vi "Ravel Index.vi"(1 "Coerce (T)":bool=TRUE, 2 "ND Index":i32[](array[numeric]), 3 "Array Shape":i32[](array[numeric])) -> (0 "Flat Index":i32)   [LabVIEW 2020, in "VIM Tools.lvlib"]
uses:
  VIM Tools.lvlib
  6fbc3370-4fe2-4f23-9844-c55be6350a4c.vi
  5715f375-2f19-42b1-8971-07d7b1a35376.vi
  f35ef6e7-f3ea-4c67-be1f-69a31266ebf5.vi
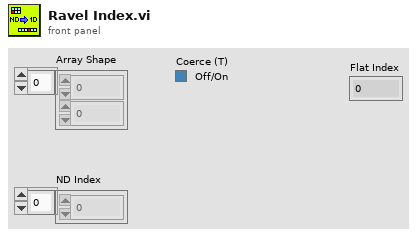
[diagram p1: front panel]
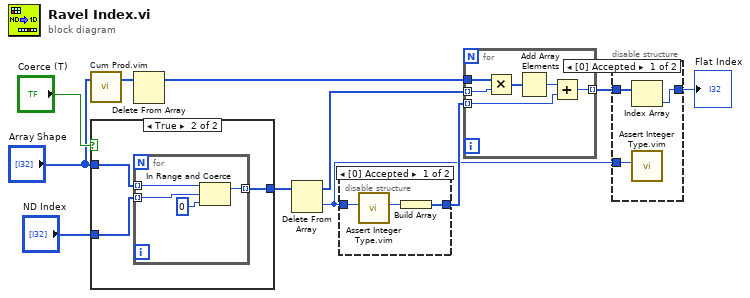
[diagram p0: block diagram]
diagram:
  n1 = call "Cum Prod.vim"("Array In"="Array Shape") -> ("Cumulated Products Out"=w10:i32[])  [unwired: 1 in, 1 out]
  n2 = case shown="True" "Coerce (T)" {
    tunnel: "ND Index" -> [w12 w15]
    tunnel: "Array Shape" -> [_ w14]
    tunnel: [w12 w13] -> w9
    frame False {
    }
    frame True {
      n3 = for {
        tunnel: w14 -> [w18] mode=indexing
        tunnel: w15 -> [w19] mode=indexing
        tunnel: [w16] -> w13 mode=indexing
        n4 = In Range and Coerce(upper limit=w18, x=w19, lower limit=0) -> (coerced(x)=w16:i32)  [unwired: 1 out]
      }
    }
  }
  n5 = Delete From Array(array=w10) -> (array with subset deleted=w8:i32[])  [unwired: 2 in, 1 out]
  n6 = Delete From Array(array=w9) -> (deleted portion=w1:i32, array with subset deleted=w7:i32[])  [unwired: 2 in]
  n7 = disable-structure shown="[0] Accepted" {
    disable-tunnel: w1 -> [w22 w23]
    disable-tunnel: [w20 w23] -> w3
    frame Enabled {
      n8 = call "Assert Integer Type.vim"("value in"=w22) -> ("value out"=w21:i32)  [unwired: 8 in]
      n9 = Build Array(w21) -> (w20:i32[])
    }
    frame Disabled {
    }
  }
  n10 = for {
    tunnel: w8 -> [w29]
    tunnel: w7 -> [w28] mode=indexing
    tunnel: w3 -> [w25] mode=indexing
    tunnel: [w24] -> w6 mode=indexing
    n11 = Multiply(x=w29, y=w28) -> (x*y=w27:i32[])
    n12 = Add Array Elements(numeric array=w27) -> (sum=w26:i32)
    n13 = Add(x=w26, y=w25) -> (x+y=w24:i32)
  }
  n14 = disable-structure shown="[0] Accepted" {
    disable-tunnel: w6 -> [w32 w33]
    disable-tunnel: [w31 w33] -> w2
    disable-tunnel: w1 -> [w30 _]
    frame Enabled {
      n15 = Index Array(array=w32) -> (element=w31:i32)  [unwired: 1 in]
      n16 = call "Assert Integer Type.vim"("value in"=w30) -> ()  [unwired: 8 in, 1 out]
    }
    frame Disabled {
    }
  }
  "Flat Index" <- w2
